vi "Outtake Controller.vi"(8 "error in":errorcluster) -> ()   [LabVIEW 2020]
doc: "This VI executes continuously carrying out the current operation and responding to updates or new operations. It will often contain the timing or control code that is difficult to place directly in TeleOp. This VI generally opens all sensors and motors and isolates the rest of the robot code from knowing how the operations are carried out."
uses:
  <vilib>/Rock Robotics/WPI/Framework/Completion Status.ctl
  Outtake Setpoints.ctl
  Outtake Operations.ctl
  <vilib>/Rock Robotics/Network Tables/NT Write Boolean.vi
panel:
  in  "Interactive Values":T1
  out "Current\nCmd":string
  in  "Buttons":cluster{"Execute Cmd":bool, "Abort Cmd":bool}
  out "Command Timing":cluster{"Start Time (ms)":u32, "Iterations":i32}
  out "Status":T3
  # "Tip: It may be helpful to observe inputs and sensor values.\nYou may also want to display tuning or debugging controls."
  # "Interactive Command: You may fill in the settings for a command\nand schedule it with the Execute button. You can observe and abort\nany command while fine tuning the code for the controller."
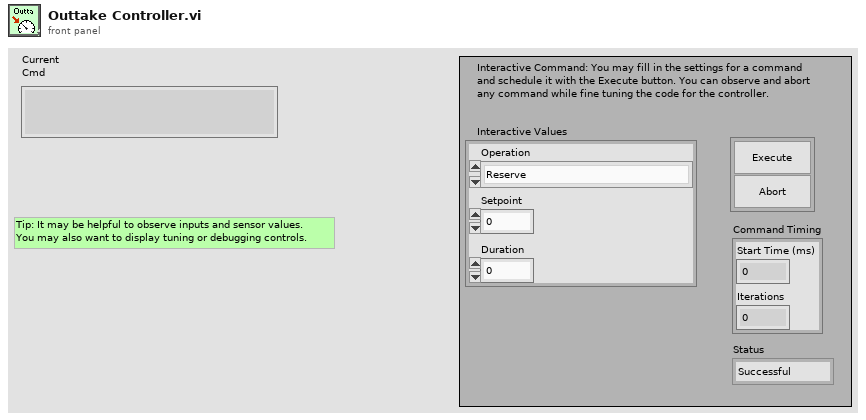
[diagram p1: front panel]
types:
  T1 = typedef "Outtake Setpoints.ctl" = cluster{"Operation":T2, "Setpoint":dbl, "Duration":dbl}
  T2 = typedef "Outtake Operations.ctl" = enum16{"Reserve", "Read Current", "Outtake Immediate", "Outtake For Time"}
  T3 = typedef "Completion Status.ctl" = enum16{"Successful", "Aborted", "Incomplete"}
  T4 = typedef "WPI_MotorControlDeviceRef.ctl" = cluster{"DeviceStatus":errorcluster, "Type":T5, "PWM":cluster{"PWM Channel":T6, "DeadBand":T7}, "CAN":cluster{"Device Number":u8, "SetOutput VI Ref":variant, "GetOutput VI Ref":variant, "Enable VI Ref":variant, "Disable VI Ref":variant, "Data":variant}, "Invert":bool, "DIO PWM":cluster{"PWM \"Enable\" Channel":T6, "DIOChannel":T8, "PWM Rate":dbl}}
  T5 = typedef "WPI_MotorControlType.ctl" = enum16{"PWM", "CAN", "DIO PWM"}
  T6 = typedef "FPGA_DIOPWMChannel.ctl" = enum8{"PWM 0", "PWM 1", "PWM 2", "PWM 3", "PWM 4", "PWM 5", "PWM 6", "PWM 7", "PWM 8", "PWM 9", "PWM MXP 0", "PWM MXP 1", "PWM MXP 2", "PWM MXP 3", "PWM MXP 4", "PWM MXP 5", "PWM MXP 6", "PWM MXP 7", "PWM MXP 8", "PWM MXP 9", "Invalid"}
  T7 = typedef "WPI_PWMDeadband.ctl" = cluster{"Name":string, "maxPositivePwm":i32, "minPositivePwm":i32, "centerPwm":i32, "maxNegativePwm":i32, "minNegativePwm":i32, "angularRange":u16}
  T8 = typedef "FPGA_DIOChannel.ctl" = enum8{"DIO 0", "DIO 1", "DIO 2", "DIO 3", "DIO 4", "DIO 5", "DIO 6", "DIO 7", "DIO 8", "DIO 9", "DIO MXP 0", "DIO MXP 1", "DIO MXP 2", "DIO MXP 3", "DIO MXP 4", "DIO MXP 5", "DIO MXP 6", "DIO MXP 7", "DIO MXP 8", "DIO MXP 9", "DIO MXP 10", "DIO MXP 11", "DIO MXP 12", "DIO MXP 13", "DIO MXP 14", "DIO MXP 15", "SPI Port CS1", "SPI Port CS2", "SPI Port CS3", "SPI Port MISO", "SPI Port MOSI", "Invalid"}
  T9 = typedef "Command Status Info.ctl" = cluster{"Name":string, "Status":T3, "notifier out":T10}
  T10 = typedef "Completion Notifier.ctl" = refnum<notifier>
  T11 = cluster{"Current Command":T1, "Command Timing":cluster{"Start Time (ms)":u32, "Iterations":i32}, "Command Arguments":cluster{"Command Info":T9, "Description":string, "Default Command":T1, "queue out":refnum<queue>, "Subsystem Name":string}}
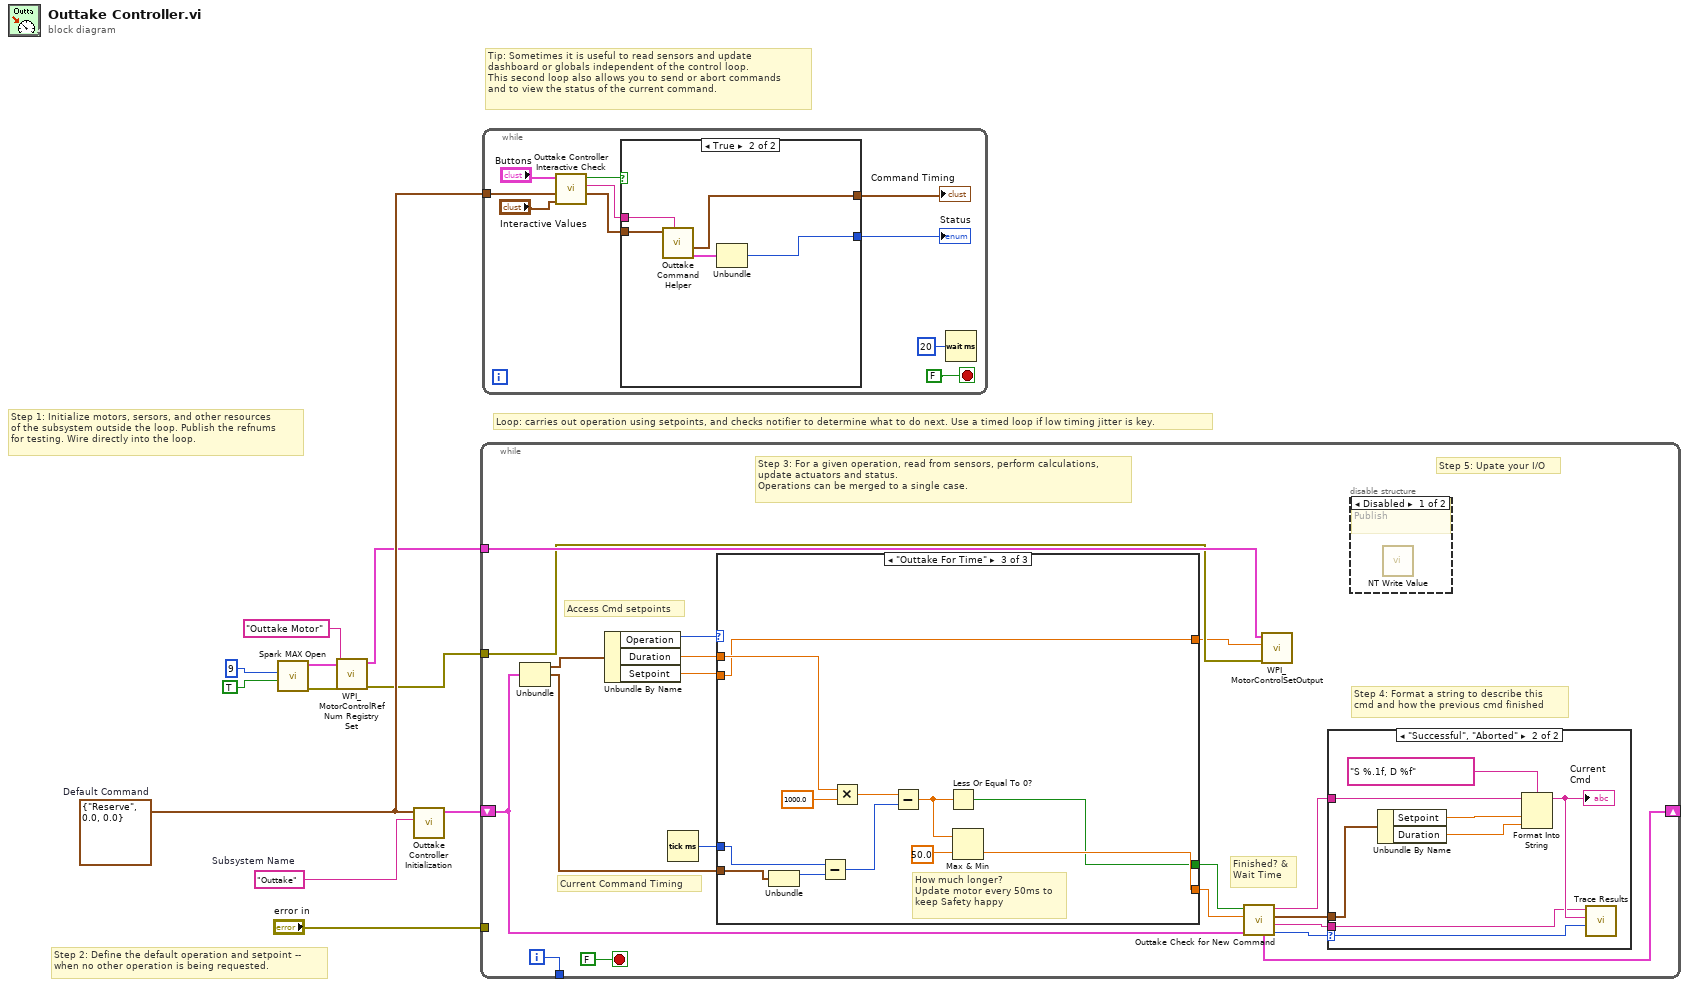
[diagram p0: block diagram]
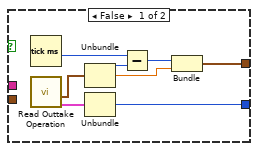
[diagram p2: hidden frame]
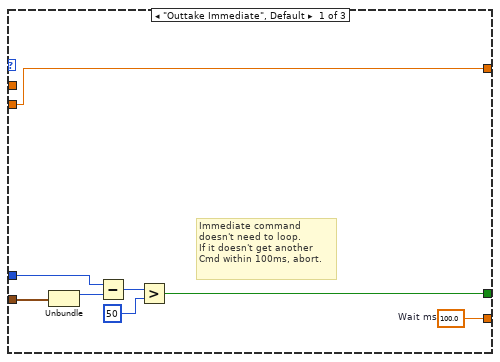
[diagram p5: hidden frame]
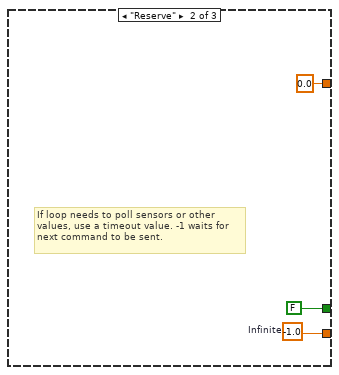
[diagram p6: hidden frame]
diagram:
  w8 = T1 {"Operation"=enum."Reserve", "Setpoint"=0.0, "Duration"=0.0}  # Default Command
  w9 = "Outtake"  # Subsystem Name
  # "Tip: Sometimes it is useful to read sensors and update\ndashboard or globals independent of the control loop.\nThis second loop also allows you to send or abort commands\nand to view the status of the current command."
  # "Step 2: Define the default operation and setpoint --\nwhen no other operation is being requested."
  # "Step 1: Initialize motors, sersors, and other resources\nof the subsystem outside the loop. Publish the refnums\nfor testing. Wire directly into the loop."
  # "Loop: carries out operation using setpoints, and checks notifier to determine what to do next. Use a timed loop if low timing jitter is key."
  n1 = call <vilib>:"Spark MAX Open.vi"("Invert"=TRUE, "Device Number"=u8 9) -> ("error out"=w3:errorcluster, "MotorControlDeviceRef"=w5:T4)  [unwired: 8 in]
  n2 = call <vilib>:"WPI_MotorControlRefNum Registry Set.vi"("error in (no error)"=w3, "refnum name"="Outtake Motor", "MotorControlDevRef"=w5) -> ("error out"=w1:errorcluster, "MotorControlDevRef"=w2:T4)  [unwired: 7 in]
  n3 = call "Outtake Controller Initialization.vi"("Subsystem Name"=w9, "Default Command"=w8) -> ("Current Command"=w10:T11)  [unwired: 9 in]
  n4 = while {
    shift-right: [w22] -> _
    shift-left: w10 -> [w15]
    tunnel: [w29] -> _
    tunnel: "error in" -> [_]
    tunnel: w2 -> [w14]
    tunnel: w1 -> [w13]
    i -> [w29]
    stop <- FALSE stop-if-true
    # "Step 5: Upate your I/O"
    # "Step 4: Format a string to describe this\ncmd and how the previous cmd finished"
    # "Current Command Timing"
    # "Access Cmd setpoints"
    # "Finished? &\nWait Time"
    # "Step 3: For a given operation, read from sensors, perform calculations,\nupdate actuators and status.\nOperations can be merged to a single case."
    n5 = Unbundle(w15) -> ("Current Command"=w28:T1, "Command Timing"=w24:cluster{"Start Time (ms)":u32, "Iterations":i32})  [unwired: 1 out]
    n6 = Unbundle By Name(w28) -> ("Operation"=w27:T2, "Duration"=w26:dbl, "Setpoint"=w23:dbl)
    n7 = Tick Count (ms)() -> (millisecond timer value=w25:u32)
    n8 = case shown="\"Outtake For Time\"" w27 {
      tunnel: [w46 w49 w55] -> w20
      tunnel: [w40 FALSE ("ignore previous (F)") w52] -> w21
      tunnel: w24 -> [w42 _ w54]
      tunnel: w26 -> [_ _ w51]
      tunnel: w25 -> [w41 _ w53]
      tunnel: w23 -> [w39 _ w50]
      tunnel: [w39 0.0 ("Setpoint") w50] -> w12
      frame "Outtake Immediate", Default {
        w46 = 100.0  # Wait ms
        # "Immediate command\ndoesn't need to loop.\nIf it doesn't get another\nCmd within 100ms, abort."
        n9 = Unbundle(w42) -> ("Start Time (ms)"=w45:u32)  [unwired: 1 out]
        n10 = Subtract(x=w41, y=w45) -> (x-y=w44:u32)
        n11 = Greater?(x=w44, y=u8 50 ("Left Motor")) -> (0:w40:bool)
      }
      frame "Reserve" {
        w49 = -1.0  # Infinite
        # "If loop needs to poll sensors or other\nvalues, use a timeout value. -1 waits for\nnext command to be sent."
      }
      frame "Outtake For Time" {
        # "How much longer?\nUpdate motor every 50ms to\nkeep Safety happy"
        n12 = Unbundle(w54) -> ("Start Time (ms)"=w58:u32)  [unwired: 1 out]
        n13 = Subtract(x=w53, y=w58) -> (x-y=w61:u32)
        n14 = Multiply(x=w51, y=1000.0) -> (x*y=w60:dbl)
        n15 = Subtract(x=w60, y=w61) -> (x-y=w57:dbl)
        n16 = Less Or Equal To 0?(x=w57) -> (x <= 0?=w52:bool)
        n17 = Max & Min(x=w57, y=50.0) -> (min(x,y)=w55:dbl)  [unwired: 1 out]
      }
    }
    n18 = call "Outtake Check for New Command.vi"("Current Command"=w15, "Wait time (ms)"=w20, "Finished?"=w21) -> ("Completion"=w16:T3, "Subsystem Name"=w17:string, "Current Command"=w18:T1, "Initial Trace String"=w19:string, "NextCommand"=w22:T11)  [unwired: 4 in]
    n19 = call <vilib>:"WPI_MotorControlSetOutput.vi"("error in (no error)"=w13, "Output"=w12, "MotorControlDevRef"=w14) -> ()  [unwired: 6 in, 3 out]
    n20 = case shown="\"Successful\", \"Aborted\"" w16 {
      selector: w16 -> [_ w38]
      tunnel: w19 -> [_ w34]
      tunnel: w18 -> [_ w35]
      tunnel: w17 -> [_ w31]
      frame "Incomplete", Default {
        # "Continuing current command"
      }
      frame "Successful", "Aborted" {
        # "Report and setup for next command"
        n21 = Unbundle By Name(w35) -> ("Setpoint"=w37:dbl, "Duration"=w32:dbl)
        n22 = Format Into String(format string="S %.1f, D %f", initial string=w34, w37, w32) -> (resulting string=w33:string)  [unwired: 1 in, 1 out]
        "Current\nCmd" <- w33
        n23 = call <vilib>:"Trace Results.vi"("Status of previous command"=w38, "Description"=w33, "Subsystem"=w31) -> ()  [unwired: 9 in]
      }
    }
    n24 = disable-structure shown="Disabled" {
      frame Disabled {
        # "Publish"
        n25 = call-poly <vilib>:"NT Write Value.vi"() -> ()  [unwired: 11 in, 1 out]
      }
      frame Enabled {
      }
    }
  }
  n26 = while {
    tunnel: w8 -> [w68]
    stop <- FALSE stop-if-true
    n27 = call "Outtake Controller Interactive Check.vi"("Interactive Command in"="Interactive Values", "Default Command"=w68, "Buttons"="Buttons") -> ("Interactive Command out"=w65:T1, "Trace String"=w66:string, "Schedule"=w67:bool)  [unwired: 6 in]
    n28 = case shown="True" w67 {
      tunnel: [w79 w84] -> w64
      tunnel: w65 -> [_ w82]
      tunnel: [w75 w80] -> w63
      tunnel: w66 -> [_ w83]
      frame False {
        n29 = Tick Count (ms)() -> (millisecond timer value=w74:u32)
        n30 = call "Read Outtake Operation.vi"() -> ("Command Info"=w72:T9, "SubSystem Data"=w73:T1)  [unwired: 9 in, 1 out]
        n31 = Unbundle(w73) -> ("Operation"=w78:T2, "Setpoint"=w76:dbl)  [unwired: 1 out]
        n32 = Unbundle(w72) -> ("Status"=w79:T3)  [unwired: 2 out]
        n33 = Subtract(x=w74, y=w78) -> (x-y=w77:u32)
        n34 = Bundle(w77, "Setpoint"=w76) -> (w75:cluster{u32, "Setpoint":dbl})  [unwired: 1 in]
      }
      frame True {
        n35 = call "Outtake Command Helper.vi"("Description"=w83, "SubSystem Data"=w82) -> ("Command Info Out"=w81:T9, "Command Timing"=w80:cluster{"Start Time (ms)":u32, "Iterations":i32})  [unwired: 7 in, 1 out]
        n36 = Unbundle(w81) -> ("Status"=w84:T3)  [unwired: 2 out]
      }
    }
    "Status" <- w64
    "Command Timing" <- w63
    n37 = Wait (ms)(milliseconds to wait=u32 20) -> ()  [unwired: 1 out]
  }
